vi "move_invader_.vi"(11 "invader_in":T1={"output cluster"={"image type"=0, "image depth"=0, "image"=[], "mask"=[], "colors"=[], "Rectangle"={"left"=0, "top"=0, "right"=0, "bottom"=0}}, "direction"=enum."right", "shot_period"=0.0, "Speed"=10, "Bounds"={"Width"=0, "Height"=0}}) -> (3 "invader_out":T1={"output cluster"={"image type"=0, "image depth"=0, "image"=[], "mask"=[], "colors"=[], "Rectangle"={"left"=0, "top"=0, "right"=0, "bottom"=0}}, "direction"=enum."right", "shot_period"=0.0, "Speed"=10, "Bounds"={"Width"=0, "Height"=0}})   [LabVIEW 2019]
uses:
  invader.ctl
  <vilib>/picture/picture.llb/imagedata.ctl
  move_dir_lr.ctl
  <vilib>/Utility/miscctls.llb/LVBoundsTypeDef.ctl
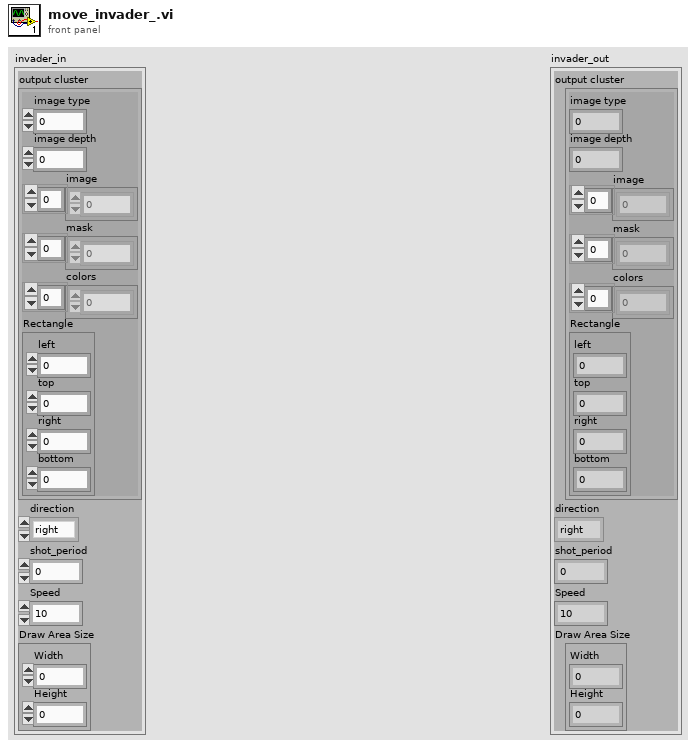
[diagram p1: front panel]
types:
  T1 = typedef "invader.ctl" = cluster{"output cluster":T2, "direction":T3, "shot_period":dbl, "Speed":i16, "Bounds":T4}
  T2 = typedef "imagedata.ctl" = cluster{"image type":i32, "image depth":i32, "image":u8[], "mask":u8[], "colors":u32[], "Rectangle":cluster{"left":i16, "top":i16, "right":i16, "bottom":i16}}
  T3 = typedef "move_dir_lr.ctl" = enum16{"right", "left"}
  T4 = typedef "LVBoundsTypeDef.ctl" = cluster{"Width":u32, "Height":u32}
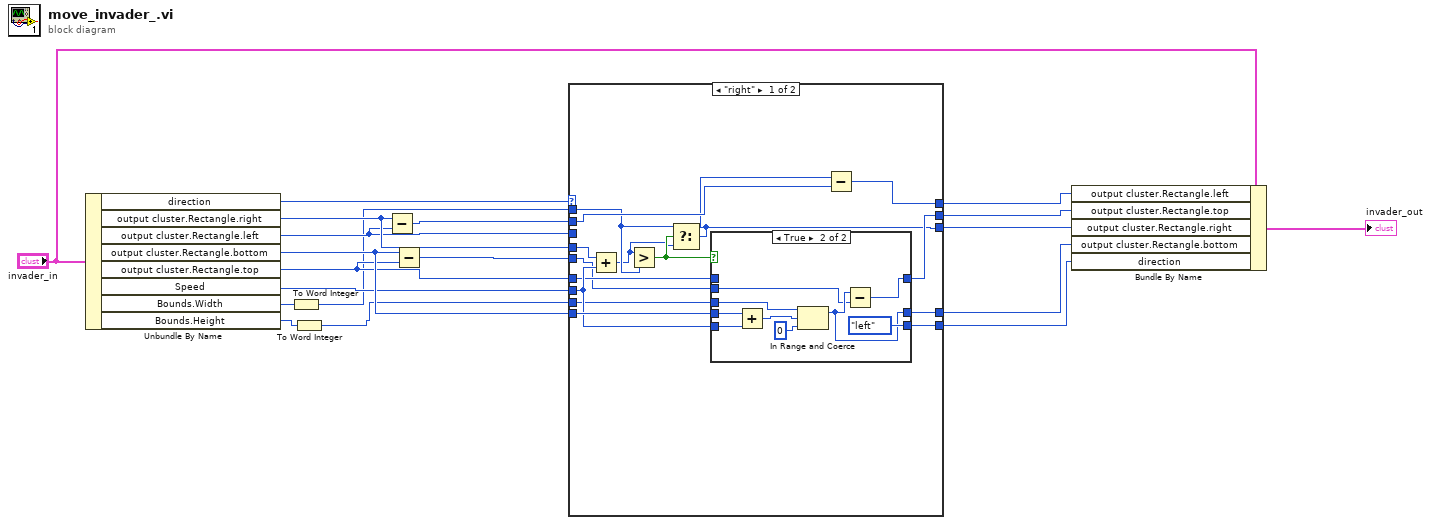
[diagram p0: block diagram]
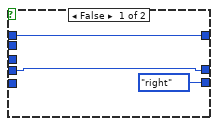
[diagram p2: hidden frame]
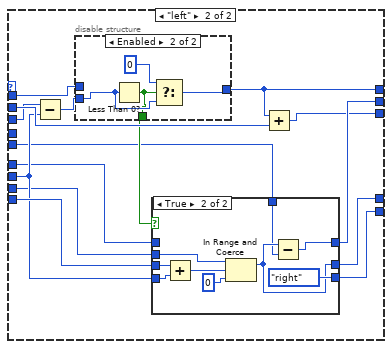
[diagram p3: hidden frame]
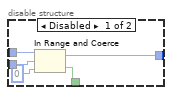
[diagram p4: hidden frame]
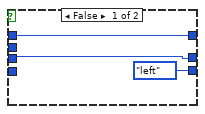
[diagram p5: hidden frame]
diagram:
  n1 = Unbundle By Name("invader_in") -> ("direction"=w19:T3, "output cluster.Rectangle.right"=w16:i16, "output cluster.Rectangle.left"=w6:i16, "output cluster.Rectangle.bottom"=w10:i16, "output cluster.Rectangle.top"=w8:i16, "Speed"=w5:i16, "Bounds.Width"=w4:u32, "Bounds.Height"=w2:u32)
  n2 = To Word Integer(number=w4) -> (16bit integer=w3:i16)
  n3 = To Word Integer(number=w2) -> (16bit integer=w1:i16)
  n4 = Subtract(x=w16, y=w6) -> (x-y=w18:i16)
  n5 = Subtract(x=w10, y=w8) -> (x-y=w17:i16)
  n6 = case shown="\"right\"" w19 {
    tunnel: w5 -> [w29 w55]
    tunnel: w18 -> [w33 w59]
    tunnel: w17 -> [w20 w47]
    tunnel: w16 -> [w34 _]
    tunnel: w3 -> [w23 w60]
    tunnel: [w21 w49] -> w13
    tunnel: [w32 w48] -> w12
    tunnel: [w31 w57] -> w11
    tunnel: w1 -> [w28 w54]
    tunnel: w10 -> [w30 w56]
    tunnel: [w27 w53] -> w9
    tunnel: w8 -> [w26 w52]
    tunnel: [w25 w51] -> w7
    tunnel: w6 -> [_ w50]
    frame "right" {
      n7 = Add(x=w34, y=w29) -> (x+y=w22:i16)
      n8 = Greater?(x=w22, y=w23) -> (0:w24:bool)
      n9 = Select(t=w23, s=w24, f=w22) -> (s? t:f=w21:i16)
      n10 = case shown="True" w24 {
        tunnel: [move_dir_lr."right" ("direction") move_dir_lr."left" ("direction")] -> w31
        tunnel: w30 -> [w36 w45]
        tunnel: w29 -> [_ w44]
        tunnel: w28 -> [_ w40]
        tunnel: [w36 w41] -> w27
        tunnel: w26 -> [w35 _]
        tunnel: [w35 w39] -> w25
        tunnel: w20 -> [_ w38]
        frame False {
        }
        frame True {
          n11 = Add(x=w45, y=w44) -> (x+y=w43:i16)
          n12 = In Range and Coerce(upper limit=w40, x=w43, lower limit=i16 0) -> (coerced(x)=w41:i16)  [unwired: 1 out]
          n13 = Subtract(x=w41, y=w38) -> (x-y=w39:i16)
        }
      }
      n14 = Subtract(x=w21, y=w33) -> (x-y=w32:i16)
    }
    frame "left" {
      n15 = Subtract(x=w50, y=w55) -> (x-y=w61:i16)
      n16 = disable-structure shown="Enabled" {
        disable-tunnel: w61 -> [w66 w69]
        disable-tunnel: w60 -> [w65 _]
        disable-tunnel: [w63 w67] -> w58
        disable-tunnel: [w62 w68] -> w48
        frame Disabled {
          n17 = In Range and Coerce(upper limit=w65, x=w66, lower limit=i16 0) -> (coerced(x)=w62:i16, In Range?=w63:bool)
        }
        frame Enabled {
          n18 = Less Than 0?(x=w69) -> (x < 0?=w67:bool)
          n19 = Select(t=i16 0 ("lower limit"), s=w67, f=w69) -> (s? t:f=w68:i16)
        }
      }
      n20 = case shown="True" w58 {
        tunnel: [move_dir_lr."left" ("direction") move_dir_lr."right" ("direction")] -> w57
        tunnel: w56 -> [w72 w81]
        tunnel: w55 -> [_ w80]
        tunnel: w54 -> [_ w76]
        tunnel: [w72 w77] -> w53
        tunnel: w52 -> [w71 _]
        tunnel: [w71 w75] -> w51
        tunnel: w47 -> [_ w74]
        frame False {
        }
        frame True {
          n21 = Add(x=w81, y=w80) -> (x+y=w79:i16)
          n22 = In Range and Coerce(upper limit=w76, x=w79, lower limit=i16 0) -> (coerced(x)=w77:i16)  [unwired: 1 out]
          n23 = Subtract(x=w77, y=w74) -> (x-y=w75:i16)
        }
      }
      n24 = Add(x=w48, y=w59) -> (x+y=w49:i16)
    }
  }
  n25 = Bundle By Name(cluster="invader_in", "output cluster.Rectangle.left"=w12, "output cluster.Rectangle.top"=w7, "output cluster.Rectangle.right"=w13, "output cluster.Rectangle.bottom"=w9, "direction"=w11) -> (→"invader_out":T1)
